vi "Build Component Value Array.vi"(6 "Component Name Array":string[](array[string]), 7 "Filter Configuration Array":refnum<class "Base Filter.lvclass">[](array[class]), 8 "error in (no error)":errorcluster, 10 "Display Data in":T1, 11 "Standard Display Configuration in":refnum<class "Standard Display Configuration.lvclass">) -> (0 "error out":errorcluster, 2 "Display Data out":T1)   [LabVIEW 2016, in "Assert API Components.lvlib" / "Assert Display.lvlib" / "Main Display.lvlib" / "Standard Display Configuration.lvclass"]
doc: "Gets the array of component values as required by the display side of the application"
uses:
  Standard Display Configuration.lvclass
  Assert Display/Assert Display.lvlib
  Assert API Components/Filter Configurations/Base Filter.lvclass
  Main Display/Display Colours.ctl
  Main Display.lvlib
  Components/Display Data.ctl
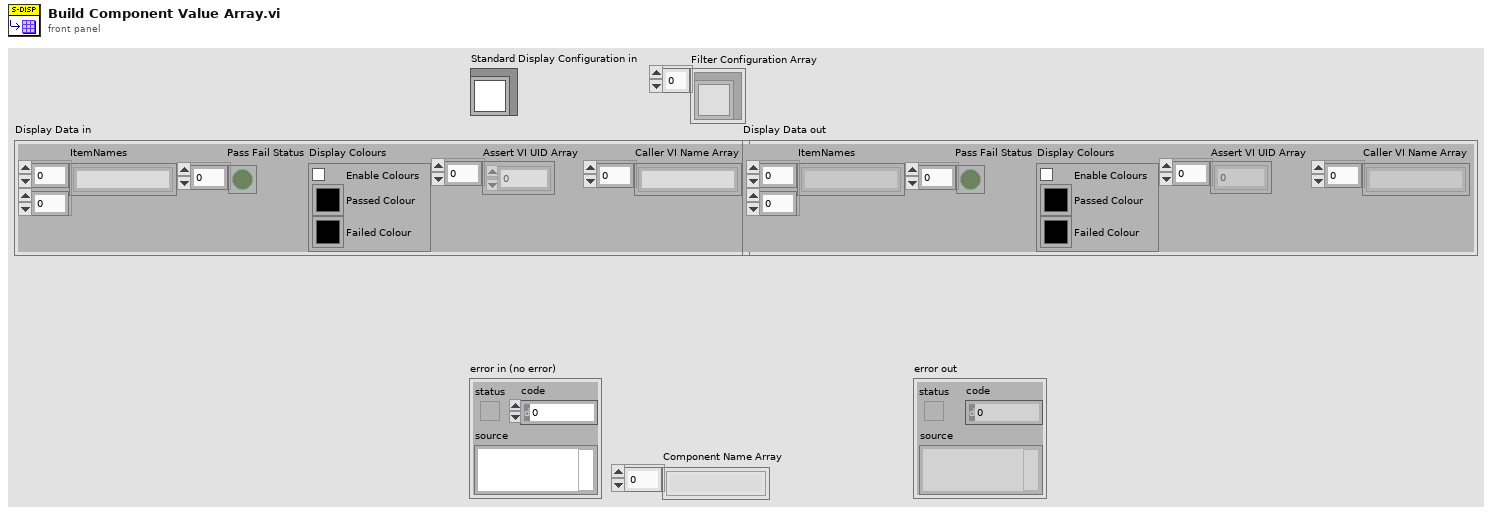
[diagram p1: front panel]
types:
  T1 = typedef "Assert API Components.lvlib/Assert Display.lvlib/Main Display.lvlib/Display Data.ctl" = cluster{"ItemNames":string[][], "Pass Fail Status":bool[], "Display Colours":T2, "Assert VI UID Array":i32[], "Caller VI Name Array":string[]}
  T2 = typedef "Assert API Components.lvlib/Assert Display.lvlib/Main Display.lvlib/Display Colours.ctl" = cluster{"Enable Colours":bool, "Passed Colour":u32, "Failed Colour":u32}
  T3 = typedef "Assert API Components.lvlib/Message Data.ctl" = cluster{"Data Value":variant, "Last Update":timestamp, "Comment":string, "Evaluation String":string, "Status":bool, "Assert Name":string, "Failure Action":T4, "Assert VI Name":string, "Calling VI Name":string, "Assert VI UID":i32, "Top Level VI Name":string, "Assert Build Timestamp":timestamp, "Assert Builder User Name":string, "Data Type":string, "IP Address":string}
  T4 = typedef "Assert API Components.lvlib/Failure Actions.ctl" = enum16{"None", "Log To File", "Pause Execution", "Abort Execution"}
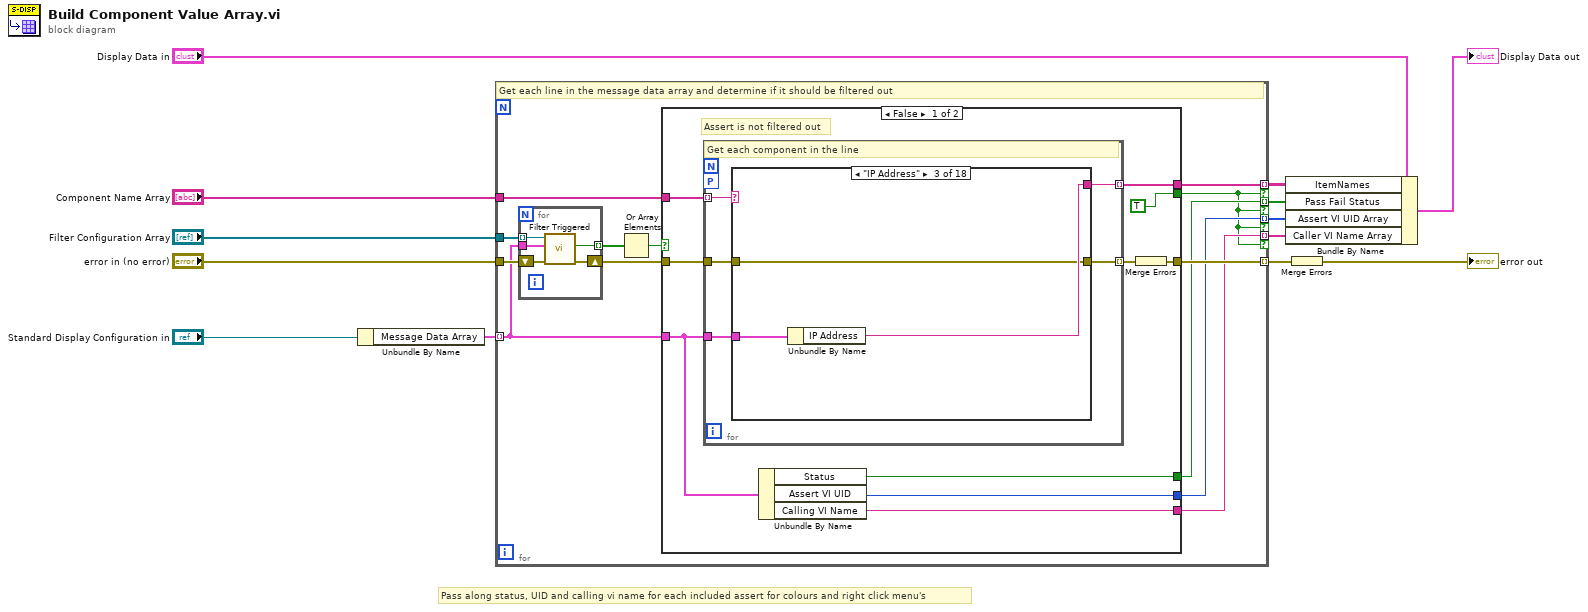
[diagram p0: block diagram]
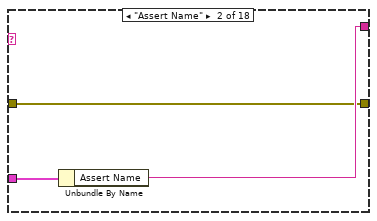
[diagram p3: hidden frame]
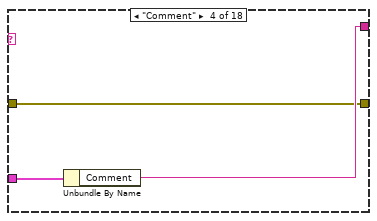
[diagram p4: hidden frame]
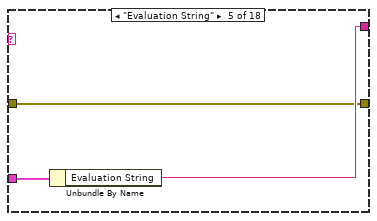
[diagram p5: hidden frame]
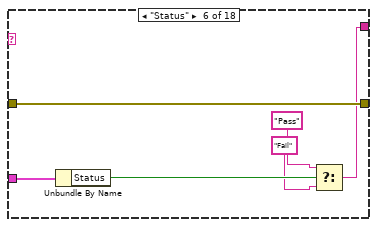
[diagram p6: hidden frame]
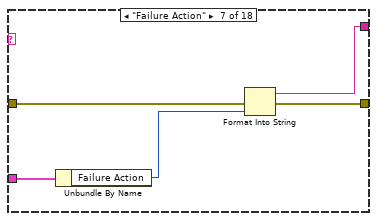
[diagram p7: hidden frame]
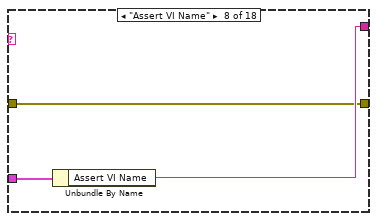
[diagram p8: hidden frame]
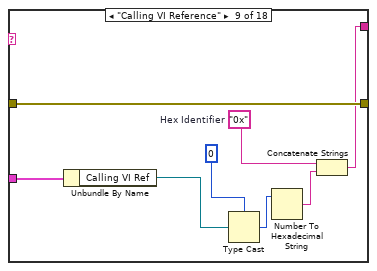
[diagram p9: hidden frame]
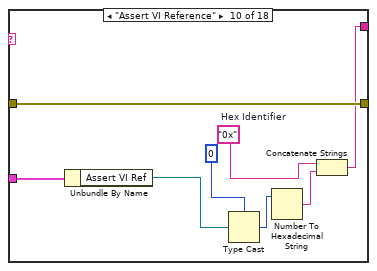
[diagram p10: hidden frame]
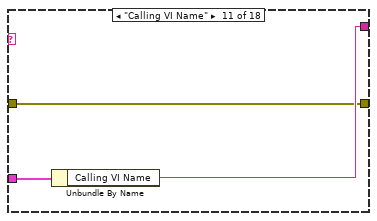
[diagram p11: hidden frame]
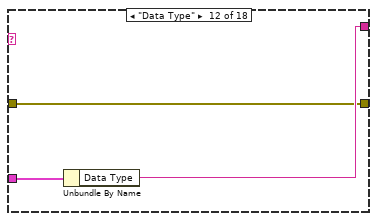
[diagram p12: hidden frame]
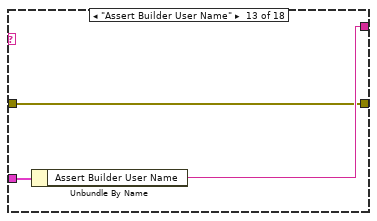
[diagram p13: hidden frame]
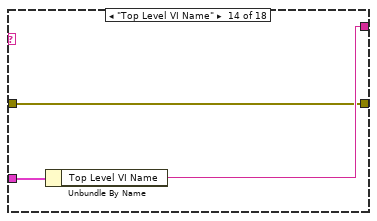
[diagram p14: hidden frame]
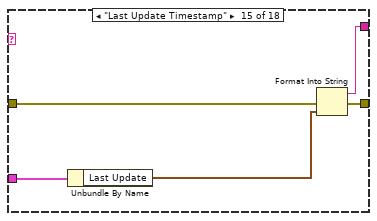
[diagram p15: hidden frame]
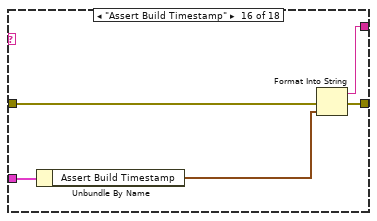
[diagram p16: hidden frame]
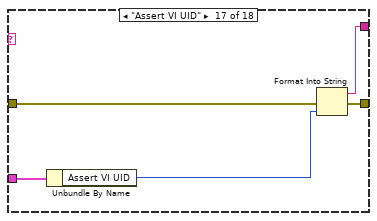
[diagram p17: hidden frame]
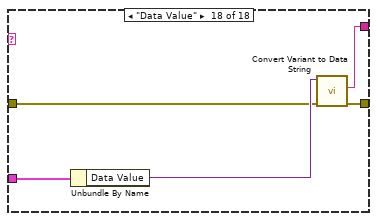
[diagram p18: hidden frame]
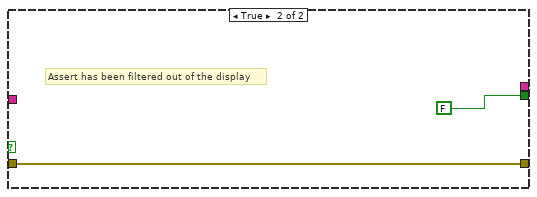
[diagram p19: hidden frame]
diagram:
  # "Pass along status, UID and calling vi name for each included assert for colours and right click menu's"
  n1 = Unbundle By Name("Standard Display Configuration in") -> ("Message Data Array"=w9:T3[])
  n2 = for {
    tunnel: "Component Name Array" -> [w26]
    tunnel: w9 -> [w18] mode=indexing
    tunnel: [w24] -> w6 mode=indexing if=w14
    tunnel: "error in (no error)" -> [w25]
    tunnel: [w23] -> w11 mode=indexing
    tunnel: [w22] -> w4 mode=indexing if=w14
    tunnel: [w21] -> w3 mode=indexing if=w14
    tunnel: "Filter Configuration Array" -> [w19]
    tunnel: [w15] -> w1 mode=indexing if=w14
    # "Get each line in the message data array and determine if it should be filtered out"
    n3 = for {
      shift-right: [w122] -> w20
      shift-left: w25 -> [w123]
      tunnel: w19 -> [w121] mode=indexing
      tunnel: w18 -> [w120]
      tunnel: [w119] -> w17 mode=indexing
      n4 = call-dynamic "Filter Triggered.vi"("error in (no error)"=w123, "Assert Message"=w120, "Base Filter in"=w121) -> ("error out"=w122:errorcluster, "Filtered"=w119:bool)  [unwired: 7 in]
    }
    n5 = Or Array Elements(Boolean array=w17) -> (logical OR=w16:bool)
    n6 = case shown="False" w16 {
      tunnel: w26 -> [w36 _]
      tunnel: [w34 _] -> w24
      tunnel: [w33 w118] -> w23
      tunnel: [w32 _] -> w22
      tunnel: [w31 _] -> w21
      tunnel: w20 -> [w30 w118]
      tunnel: w18 -> [w29 _]
      tunnel: [TRUE FALSE] -> w14
      tunnel: [w27 _] -> w15
      frame False {
        # "Assert is not filtered out"
        n7 = for {
          tunnel: w36 -> [w41] mode=indexing
          tunnel: w29 -> [w38]
          tunnel: [w37] -> w34 mode=indexing
          tunnel: w30 -> [w40]
          tunnel: [w39] -> w35 mode=indexing
          workers-P: _ -> [_]
          # "Get each component in the line"
          n8 = case shown="\"IP Address\"" w41 {
            tunnel: w38 -> [_ w45 w48 w51 w54 w60 w65 w68 w76 w84 w87 w90 w93 w96 w101 w106 w111 w116]
            tunnel: [_ w44 w47 w50 w53 w55 w61 w67 w70 w78 w86 w89 w92 w95 w97 w102 w107 w115] -> w37
            tunnel: w40 -> [w42 w43 w46 w49 w52 w59 w64 w66 w75 w79 w85 w88 w91 w94 w100 w105 w110 w112]
            tunnel: [w42 w43 w46 w49 w52 w59 w63 w66 w75 w79 w85 w88 w91 w94 w99 w104 w109 w114] -> w39
            frame Default {
            }
            frame "Assert Name" {
              n9 = Unbundle By Name(w45) -> ("Assert Name"=w44:string)
            }
            frame "IP Address" {
              n10 = Unbundle By Name(w48) -> ("IP Address"=w47:string)
            }
            frame "Comment" {
              n11 = Unbundle By Name(w51) -> ("Comment"=w50:string)
            }
            frame "Evaluation String" {
              n12 = Unbundle By Name(w54) -> ("Evaluation String"=w53:string)
            }
            frame "Status" {
              n13 = Unbundle By Name(w60) -> ("Status"=w58:bool)
              n14 = Select(t="Pass", s=w58, f="Fail") -> (s? t:f=w55:string)
            }
            frame "Failure Action" {
              n15 = Unbundle By Name(w65) -> ("Failure Action"=w62:T4)
              n16 = Format Into String(error in=w64, w62) -> (resulting string=w61:string, error out=w63:errorcluster)  [unwired: 2 in]
            }
            frame "Assert VI Name" {
              n17 = Unbundle By Name(w68) -> ("Assert VI Name"=w67:string)
            }
            frame "Calling VI Reference" {
              w69 = "0x"  # Hex Identifier
              n18 = Unbundle By Name(w76) -> ("Calling VI Ref"=w72:refnum<vi>)
              n19 = Type Cast(type=u32 0, x=w72) -> (*(type *) &x=w73:u32)
              n20 = Number To Hexadecimal String(2:w73) -> (0:w71:string)  [unwired: 1 in]
              n21 = Concatenate Strings(w69, w71) -> (w70:string)
            }
            frame "Assert VI Reference" {
              w77 = "0x"  # Hex Identifier
              n22 = Unbundle By Name(w84) -> ("Assert VI Ref"=w82:refnum<vi>)
              n23 = Type Cast(type=u32 0, x=w82) -> (*(type *) &x=w80:u32)
              n24 = Number To Hexadecimal String(2:w80) -> (0:w81:string)  [unwired: 1 in]
              n25 = Concatenate Strings(w77, w81) -> (w78:string)
            }
            frame "Calling VI Name" {
              n26 = Unbundle By Name(w87) -> ("Calling VI Name"=w86:string)
            }
            frame "Data Type" {
              n27 = Unbundle By Name(w90) -> ("Data Type"=w89:string)
            }
            frame "Assert Builder User Name" {
              n28 = Unbundle By Name(w93) -> ("Assert Builder User Name"=w92:string)
            }
            frame "Top Level VI Name" {
              n29 = Unbundle By Name(w96) -> ("Top Level VI Name"=w95:string)
            }
            frame "Last Update Timestamp" {
              n30 = Unbundle By Name(w101) -> ("Last Update"=w98:timestamp)
              n31 = Format Into String(error in=w100, w98) -> (resulting string=w97:string, error out=w99:errorcluster)  [unwired: 2 in]
            }
            frame "Assert Build Timestamp" {
              n32 = Unbundle By Name(w106) -> ("Assert Build Timestamp"=w103:timestamp)
              n33 = Format Into String(error in=w105, w103) -> (resulting string=w102:string, error out=w104:errorcluster)  [unwired: 2 in]
            }
            frame "Assert VI UID" {
              n34 = Unbundle By Name(w111) -> ("Assert VI UID"=w108:i32)
              n35 = Format Into String(error in=w110, w108) -> (resulting string=w107:string, error out=w109:errorcluster)  [unwired: 2 in]
            }
            frame "Data Value" {
              n36 = Unbundle By Name(w116) -> ("Data Value"=w113:variant)
              n37 = call "Convert Variant to Data String.vi"("error in (no error)"=w112, "Data Value"=w113) -> ("error out"=w114:errorcluster, "Data Value String"=w115:string)  [unwired: 8 in]
            }
          }
        }
        n38 = Unbundle By Name(w29) -> ("Status"=w32:bool, "Assert VI UID"=w31:i32, "Calling VI Name"=w27:string)
        n39 = Merge Errors(w35) -> (w33:errorcluster)
      }
      frame True {
        # "Assert has been filtered out of the display"
      }
    }
  }
  n40 = Bundle By Name(cluster="Display Data in", "ItemNames"=w6, "Pass Fail Status"=w4, "Assert VI UID Array"=w3, "Caller VI Name Array"=w1) -> (→"Display Data out":T1)
  n41 = Merge Errors(w11) -> (→"error out":errorcluster)
